vi "Shooter Immediate Wrapper.vi"() -> ()   [LabVIEW 2019]
uses:
  Implementation/Shooter Operations.ctl
panel:
  in  "Operation":T1=enum."Immediate"
  in  "Manual Addition":dbl
  in  "Hood":dbl
  in  "AA?":bool
  in  "Flywheel":dbl
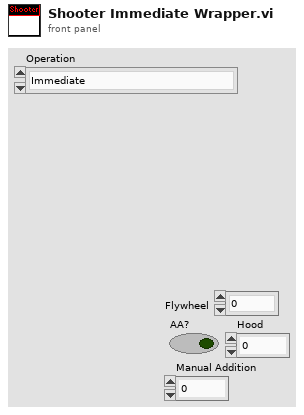
[diagram p1: front panel]
types:
  T1 = typedef "Shooter Operations.ctl" = enum16{"Reserve", "Read Current", "Immediate", "Shoot"}
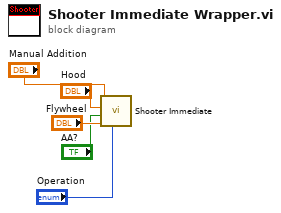
[diagram p0: block diagram]
diagram:
  n1 = call "Shooter Immediate.vi"("Operation"="Operation", "Flywheel"="Flywheel", "AA?"="AA?", "Hood"="Hood", "Manual Addition"="Manual Addition") -> ()  [unwired: 7 in]
